vi "TwTpsConnect2.vi"(1 "type":i32, 2 "ip":string, 3 "error in (no error)":errorcluster) -> (0 "error out":errorcluster)   [LabVIEW 2009]
uses:
  Release_Build/TofDaqDll.dll
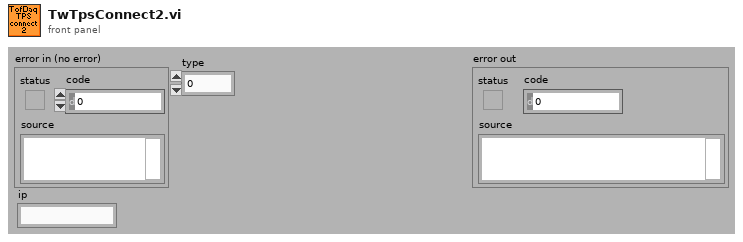
[diagram p1: front panel]
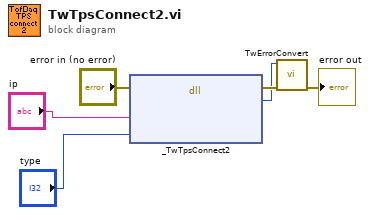
[diagram p0: block diagram]
diagram:
  n1 = dll-call lib="C:/src/TofDaq/Release_Build/TofDaqDll.dll" fn="_TwTpsConnect2"(error in="error in (no error)", "ip"="ip", "type"="type") -> (error out=w5:errorcluster, "TwRetVal"=w3:i32)  [unwired: 2 in, 3 out]
  n2 = call "TwErrorConvert.vi"("error in (no error)"=w5, "error code"=w3) -> ("error out"=→"error out":errorcluster)  [unwired: 9 out]
